vi "Startup.vi"(7 "Application":refnum<class "Application.lvclass">, 8 "error in (no error)":errorcluster, 10 "Config":refnum<class "Config.lvclass">, 11 "DAQ_Engine in":refnum<class "DAQ_Engine.lvclass">) -> (0 "error out":errorcluster, 3 "DAQ_Engine out":refnum<class "DAQ_Engine.lvclass">, 5 "Application out":refnum<class "Application.lvclass">)   [LabVIEW 2019, in "DAQ_Engine.lvclass"]
doc: "Developed by Kevin Thompson\nkevin@thompsonengineering.net\n\nCopyright 2018\nThompson Engineering, LLC"
uses:
  DAQ_Engine.lvclass
  Config/Config.lvclass
  Application/Application.lvclass
  DataTypes/Dependency--cluster.ctl
  Application/Application.lvclass/Application.ctl
  DAQ_Engine.lvclass/DAQ_Engine.ctl
  Application/Accessors/Get RawDaqDataQRef.vi
  Accessors/Set Dependency.vi
  Accessors/Set Settings.vi
  Accessors/Set MeasSettings.vi
  Accessors/Set InverterDataAcqMode.vi
  Accessors/Set RawDaqDataQRef.vi
  Config/Accessors/Get DAQ Settings.vi
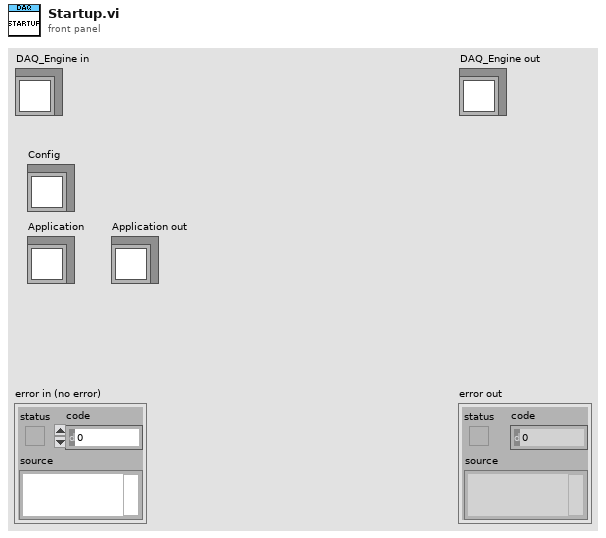
[diagram p1: front panel]
types:
  T1 = typedef "DAQ_Engine.lvclass/Dependency--cluster.ctl" = cluster{"Config":refnum<class "Config.lvclass">}
  T2 = typedef "DAQ_Engine.lvclass/Settings--cluster.ctl" = cluster{"Simulation":bool, "Initial ErrReporting setting":i32, "Initial Measurement settings":T3, "Acquisition mode":T4, "DemoMode":bool, "RIO Device":string}
  T3 = typedef "Measurement Config--cluster.ctl" = cluster{"Data Rate 9775":dbl, "Data Rate 9215":dbl, "Samples RMS 9215":u32, "Samples RMS 9775":u32}
  T4 = typedef "Acquisition Mode--cluster.ctl" = enum16{"3phase", "Single"}
  T5 = typedef "RawDAQDataQRef--cluster.ctl" = refnum<queue>
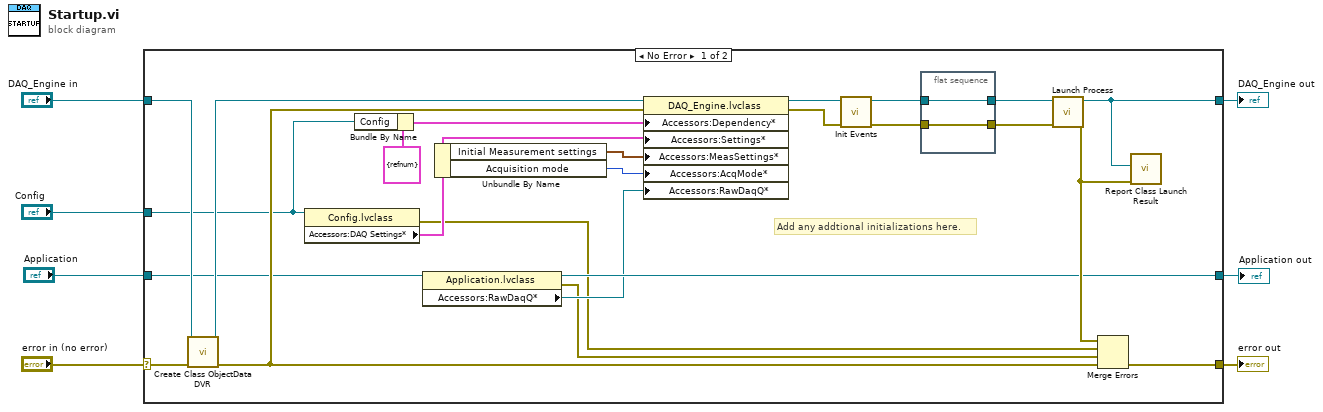
[diagram p0: block diagram]
diagram:
  n1 = case shown="No Error" "error in (no error)" {
    selector: "error in (no error)" -> [w31 w36]
    tunnel: [w24 w36] -> w6
    tunnel: [w17 w35] -> w4
    tunnel: "DAQ_Engine in" -> [w29 w35]
    tunnel: "Config" -> [w15 _]
    tunnel: "Application" -> [w18 w34]
    tunnel: [w11 w34] -> w1
    frame No Error {
      # "Add any addtional initializations here."
      n2 = call "Create Class ObjectData DVR.vi"("error in (no error)"=w31, "DAQ_Engine in"=w29) -> ("error out"=w21:errorcluster, "DAQ_Engine out"=w28:refnum<class "DAQ_Engine.lvclass">)  [unwired: 8 in]
      n3 = property class="Config.lvclass"(reference=w15) -> (error out=w8:errorcluster, "Accessors:DAQ Settings*"=w14:T2)  [unwired: 1 in, 1 out]
      n4 = Bundle By Name(cluster=T1 {"Config"=refnum} ("Dependency"), "Config"=w15) -> (w19:T1)
      n5 = property class="Application.lvclass"(reference=w18) -> (reference out=w11:refnum<class "Application.lvclass">, error out=w9:errorcluster, "Accessors:RawDaqQ*"=w10:T5)  [unwired: 1 in]
      n6 = Unbundle By Name(w14) -> ("Initial Measurement settings"=w13:T3, "Acquisition mode"=w12:T4)
      n7 = property class="DAQ_Engine.lvclass"(reference=w28, error in=w21, "Accessors:Dependency*"=w19, "Accessors:Settings*"=w14, "Accessors:MeasSettings*"=w13, "Accessors:AcqMode*"=w12, "Accessors:RawDaqQ*"=w10) -> (reference out=w30:refnum<class "DAQ_Engine.lvclass">, error out=w27:errorcluster)
      n8 = call "Init Events.vi"("error in (no error)"=w27, "DAQ_Engine in"=w30) -> ("error out"=w25:errorcluster, "DAQ_Engine out"=w26:refnum<class "DAQ_Engine.lvclass">)  [unwired: 8 in]
      n9 = flat-sequence {
        tunnel: w26 -> [w33]
        tunnel: [w33] -> w22
        tunnel: w25 -> [w32]
        tunnel: [w32] -> w23
        frame #0 {
        }
      }
      n10 = call "Launch Process.vi"("error in (no error)"=w23, "DAQ_Engine in"=w22) -> ("error out"=w16:errorcluster, "DAQ_Engine out"=w17:refnum<class "DAQ_Engine.lvclass">)  [unwired: 6 in, 2 out]
      n11 = Merge Errors(w16, w8, w9, w21) -> (w24:errorcluster)
      n12 = call "Report Class Launch Result.vi"("Object"=w17, "error in (no error)"=w16) -> ()  [unwired: 8 in, 1 out]
    }
    frame Error {
    }
  }
  "error out" <- w6
  "DAQ_Engine out" <- w4
  "Application out" <- w1
